vi "CF_FP_to_DSC.vi"(0 "str":string[](array[string]), 1 "str var":refnum<k21>[](array[refnum])=["ni.var.psp://housesoftheholy/Leiden CF900/CF_FP_STATE"], 2 "dbl":dbl[](array[numeric]), 3 "dbl var":refnum<k21>[](array[refnum])=["ni.var.psp://housesoftheholy/Leiden CF900/Leiden CF FP/CF FP P1", "ni.var.psp://housesoftheholy/Leiden CF900/Leiden CF FP/CF FP P2", "ni.var.psp://housesoftheholy/Leiden CF900/Leiden CF FP/CF FP P3", "ni.var.psp://housesoftheholy/Leiden CF900/Leiden CF FP/CF FP P4", "ni.var.psp://housesoftheholy/Leiden CF900/Leiden CF FP/CF FP P5", "ni.var.psp://housesoftheholy/Leiden CF900/Leiden CF FP/CF FP P6", "ni.var.psp://housesoftheholy/Leiden CF900/Leiden CF FP/CF FP P7", "ni.var.psp://housesoftheholy/Leiden CF900/Leiden CF FP/CF FP Flow", "ni.var.psp://housesoftheholy/Leiden CF900/Leiden CF FP/CF FP MG0", "ni.var.psp://housesoftheholy/Leiden CF900/Leiden CF FP/CF FP MG1", "ni.var.psp://housesoftheholy/Leiden CF900/Leiden CF FP/CF FP MG2", "ni.var.psp://housesoftheholy/Leiden CF900/Leiden CF FP/CF FP MG3", "ni.var.psp://housesoftheholy/Leiden CF900/Leiden CF FP/CF FP MG4", "ni.var.psp://housesoftheholy/Leiden CF900/Leiden CF FP/CF FP MG5", "ni.var.psp://housesoftheholy/Leiden CF900/Leiden CF FP/CF FP PT on", "ni.var.psp://housesoftheholy/Leiden CF900/Leiden CF FP/CF FP W_in", "ni.var.psp://housesoftheholy/Leiden CF900/Leiden CF FP/CF FP W_out", "ni.var.psp://housesoftheholy/Leiden CF900/Leiden CF FP/CF FP He", "ni.var.psp://housesoftheholy/Leiden CF900/Leiden CF FP/CF FP oil", "ni.var.psp://housesoftheholy/Leiden CF900/Leiden CF FP/CF FP P_low", "ni.var.psp://housesoftheholy/Leiden CF900/Leiden CF FP/CF FP P_high", "ni.var.psp://housesoftheholy/Leiden CF900/Leiden CF FP/CF FP PT current", "ni.var.psp://housesoftheholy/Leiden CF900/Leiden CF FP/CF FP state0", "ni.var.psp://housesoftheholy/Leiden CF900/Leiden CF FP/CF FP state1", "ni.var.psp://housesoftheholy/Leiden CF900/Leiden CF FP/CF FP state2"]) -> ()   [LabVIEW 2016]
panel:
  out "error out":errorcluster
  in  "error in (no error)":errorcluster
  # "CF FP to DSC"
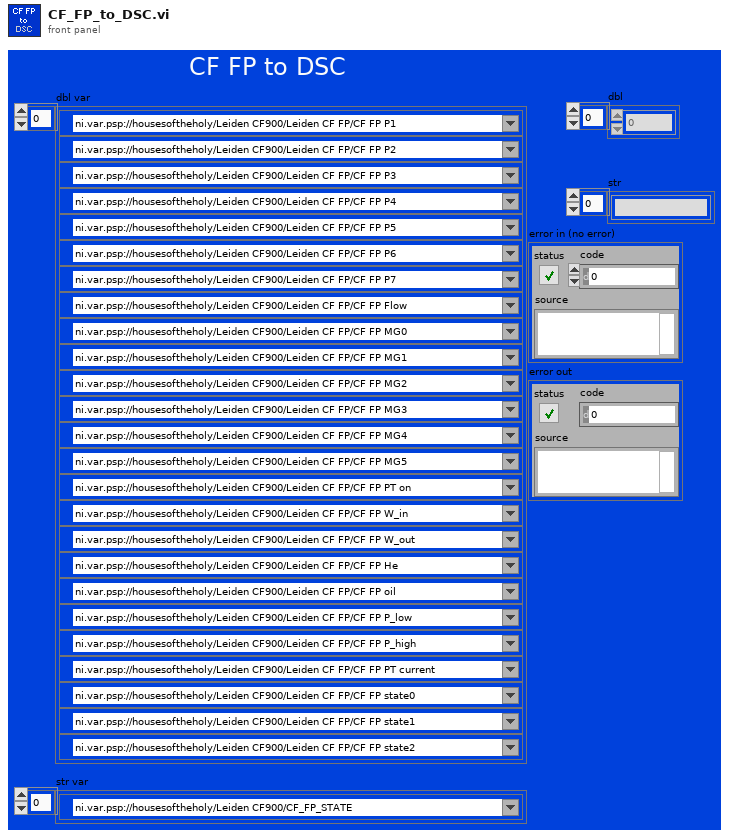
[diagram p1: front panel]
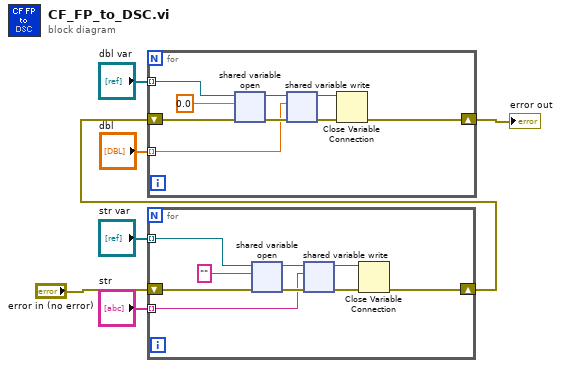
[diagram p0: block diagram]
diagram:
  n1 = for {
    tunnel: "str var" -> [w12] mode=indexing
    tunnel: "str" -> [w13] mode=indexing
    shift-right: [w10] -> w2
    shift-left: "error in (no error)" -> [w11]
    n2 = shared-variable-open(w12, w11, "") -> (w9:refnum<k21>, w15:errorcluster)  [unwired: 1 in]
    n3 = shared-variable-write(w9, w15, w13) -> (w8:refnum<k21>, w16:errorcluster)
    n4 = Close Variable Connection(8:w16, 11:w8) -> (0:w10:errorcluster)
  }
  n5 = for {
    tunnel: "dbl var" -> [w20] mode=indexing
    tunnel: "dbl" -> [w19] mode=indexing
    shift-right: [w18] -> w1
    shift-left: w2 -> [w17]
    n6 = shared-variable-open(w20, w17, 0.0) -> (w23:refnum<k21>, w24:errorcluster)  [unwired: 1 in]
    n7 = shared-variable-write(w23, w24, w19) -> (w22:refnum<k21>, w25:errorcluster)
    n8 = Close Variable Connection(8:w25, 11:w22) -> (0:w18:errorcluster)
  }
  "error out" <- w1
